vi "Validate Next State.vi"(5 "queue error in":errorcluster, 7 "error in":errorcluster, 9 "Normal State":T1, 10 "Measure Call Context in":refnum<class "Measure Call Context.lvclass">) -> (0 "error out":errorcluster, 2 "Next State":T1, 3 "measure call context out":refnum<class "Measure Call Context.lvclass">)   [LabVIEW 2025, in "Automotive Ethernet Bus Monitor.lvclass"]
uses:
  Automotive Ethernet Bus Monitor.lvclass
  Automotive Ethernet Bus Monitor.lvclass/Automotive Ethernet Bus Monitor.ctl
  <vilib>/Plug-In SDKs/Measurements/Measure Call Context/Measure Call Context.lvclass
  State.ctl
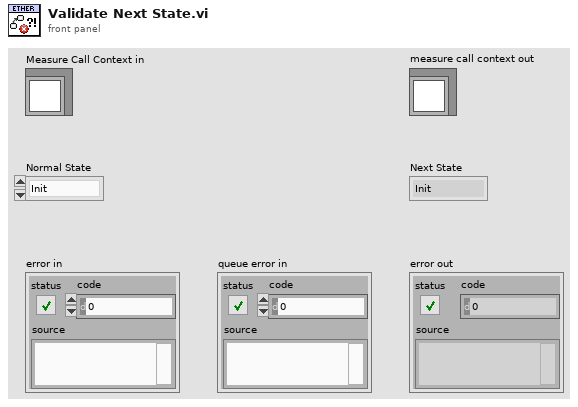
[diagram p1: front panel]
types:
  T1 = typedef "Automotive Ethernet Bus Monitor.lvclass/State.ctl" = enum16{"Init", "Execute", "Results", "Error", "Close"}
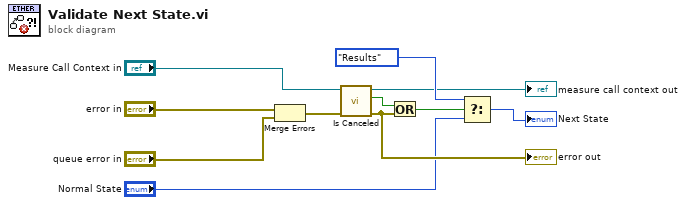
[diagram p0: block diagram]
diagram:
  n1 = Merge Errors("error in", "queue error in") -> (w4:errorcluster)
  n2 = call <vilib>:"Is Canceled.vi"("error in"=w4, "measure call context in"="Measure Call Context in") -> ("error out"=w11:errorcluster, "is canceled?"=w2:bool, "measure call context out"=→"measure call context out":refnum<class "Measure Call Context.lvclass">)  [unwired: 7 in]
  "error out" <- w11
  n3 = Or(x=w2, y=w11) -> (x .or. y?=w5:bool)
  n4 = Select(t=State."Results" ("State"), s=w5, f="Normal State") -> (s? t:f=→"Next State":T1)
